vi "Request Compatible Hardware from Client.vi"(8 "error in (no error)":errorcluster, 9 "Measurement":string, 10 "ConnectionID":string, 11 "Server Controller in":refnum<class "Server Controller.lvclass">) -> (0 "error out":errorcluster, 3 "Server Controller out":refnum<class "Server Controller.lvclass">)   [LabVIEW 2026, in "Server Controller.lvlib" / "Server Controller.lvclass"]
uses:
  Server Controller.lvclass
  C:/Users/E2013170/Documents/GitHub/Measurement-Utility-Reference/source/framework/Controller/Controller.lvclass
  framework/Controller/Messages/Find Devices of Specified Type Msg/Find Devices of Specified Type Msg.lvclass
  C:/Program Files/National Instruments/LabVIEW 2026/vi.lib/ActorFramework/Message/Message.lvclass
  framework/Controller/Messages/Find Devices of Specified Type Msg/Find Devices of Specified Type Msg.lvclass/Find Devices of Specified Type Msg.ctl
  framework/Measurement Actor/Measurement.lvclass
  recovery/packages/ni_lib_linked_network_actor-1.2.0.19-9492AF5A82/File Group 0/vi.lib/NI/Actors/Linked Network Actor/Linked Network Actor Messages/Transmit Network Message Msg/Transmit Network Message Msg.lvclass
  framework/Controller/Controller.lvclass
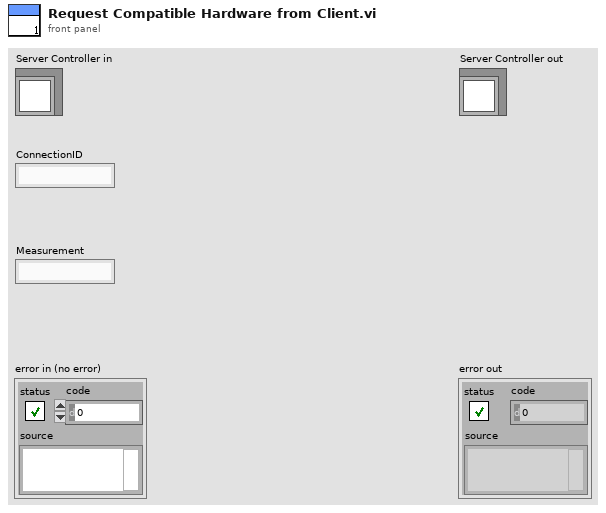
[diagram p1: front panel]
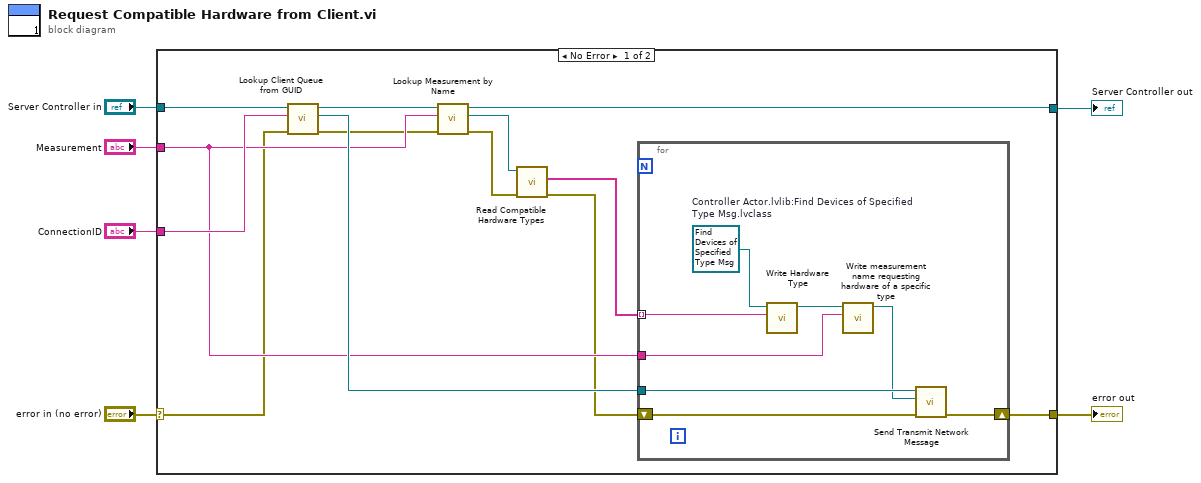
[diagram p0: block diagram]
diagram:
  n1 = case shown="No Error" "error in (no error)" {
    selector: "error in (no error)" -> [w11 w29]
    tunnel: [w7 w29] -> w5
    tunnel: [w14 w28] -> w3
    tunnel: "Server Controller in" -> [w19 w28]
    tunnel: "ConnectionID" -> [w18 _]
    tunnel: "Measurement" -> [w13 _]
    frame No Error {
      n2 = call "Lookup Client Queue from GUID.vi"("error in (no error)"=w11, "GUID"=w18, "Server Controller in"=w19) -> ("error out"=w10:errorcluster, "Caller-To-Actor Enqueuer"=w17:refnum<class "Message Enqueuer.lvclass">, "Server Controller out"=w15:refnum<class "Server Controller.lvclass">)  [unwired: 5 in, 1 out]
      n3 = call "Lookup Measurement by Name.vi"("error in (no error)"=w10, "Measurement Name"=w13, "Controller in"=w15) -> ("error out"=w9:errorcluster, "Measurement.lvclass"=w16:refnum<class "Measurement.lvclass">, "Controller out"=w14:refnum<class "Server Controller.lvclass">)  [unwired: 5 in, 1 out]
      n4 = call-dynamic "Read Compatible Hardware Types.vi"("error in (no error)"=w9, "Measurement in"=w16) -> ("error out"=w8:errorcluster, "Compatible Hardware Types"=w12:string[])  [unwired: 7 in, 1 out]
      n5 = for {
        tunnel: w17 -> [w27]
        tunnel: w13 -> [w20]
        tunnel: w12 -> [w25] mode=indexing
        shift-right: [w23] -> w7
        shift-left: w8 -> [w24]
        w26 = refnum<class "Find Devices of Specified Type Msg.lvclass"> refnum  # Controller Actor.lvlib:Find Devices of Specified Type Msg.lvclass
        n6 = call "Write Hardware Type.vi"("Hardware Type"=w25, "Find Devices of Specified Type Msg in"=w26) -> ("Find Devices of Specified Type Msg out"=w22:refnum<class "Find Devices of Specified Type Msg.lvclass">)  [unwired: 9 in]
        n7 = call "Write measurement name requesting hardware of a specific type.vi"("Measurement Name"=w20, "Find Devices of Specified Type Msg in"=w22) -> ("Find Devices of Specified Type Msg out"=w21:refnum<class "Find Devices of Specified Type Msg.lvclass">)  [unwired: 9 in]
        n8 = call "Send Transmit Network Message.vi"("error in (no error)"=w24, "Message"=w21, "Message Enqueuer"=w27) -> ("error out"=w23:errorcluster)  [unwired: 7 in, 1 out]
      }
    }
    frame Error {
    }
  }
  "error out" <- w5
  "Server Controller out" <- w3
